vi "Close Session.vi"(8 "error in":errorcluster, 10 "Session In":T1, 11 "Text Session":refnum<class "FPGA Serial Session.lvclass">) -> (0 "error out":errorcluster, 2 "Session Out":T1)   [LabVIEW 2014, in "FPGA Serial Session.lvclass"]
uses:
  FPGA Serial Session.lvclass
  <userlib>/_Session Fwk/Typedefs/Session Handle.ctl
  <userlib>/_Session Fwk/Session - Root.lvclass
  Raw FPGA/FPGA Session.lvclass
  FPGA Serial Session.lvclass/FPGA Serial Session.ctl
  Read fpgaSession.vi
  Reusable/Session APIs/Text Communication/Text Device Session.lvclass
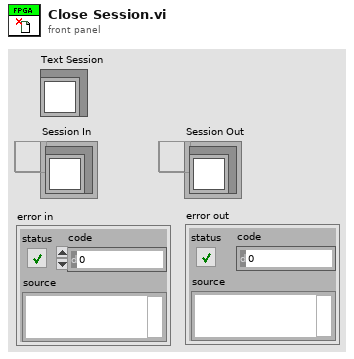
[diagram p1: front panel]
types:
  T1 = typedef "Session - Root.lvclass/Session Handle.ctl" = refnum<data-value>
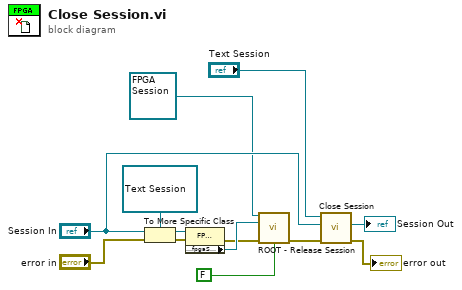
[diagram p0: block diagram]
diagram:
  n1 = To More Specific Class(target class=refnum<data-value> refnum ("Session In"), reference="Session In", error in="error in") -> (specific class reference=w9:refnum<data-value>, error out=w7:errorcluster)
  n2 = property class="FPGA Serial Session"(reference=w9, error in=w7) -> (error out=w3:errorcluster, "Accessors:fpgaSession"=w6:T1)  [unwired: 1 out]
  n3 = call <userlib>:"ROOT - Release Session.vi"("OBJ - Session in"=refnum<class "FPGA Session.lvclass"> refnum ("FPGA Session"), "Session Handle in"=w6, "error in (no error)"=w3, "force destroy? (F)"=FALSE) -> ("error out"=w2:errorcluster)  [unwired: 9 in, 2 out]
  n4 = call-parent "Close Session.vi"("error in (no error)"=w2, "Session In"="Session In", "Text Session"="Text Session") -> ("error out"=→"error out":errorcluster, "Session Out"=→"Session Out":T1)  [unwired: 7 in]
